vi "DRIVE_STRAIGHT_CAM.vi"(10 "argv":string[](array[string]), 11 "args":u8) -> ()   [LabVIEW 2011]
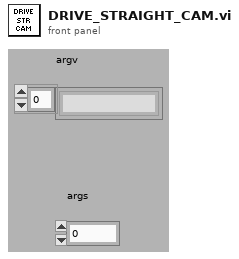
[diagram p1: front panel]
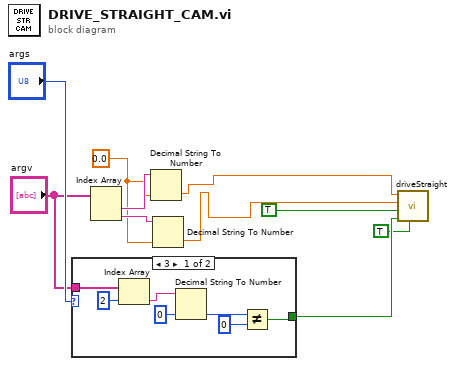
[diagram p0: block diagram]
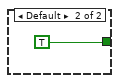
[diagram p2: hidden frame]
diagram:
  w8 = 0.0
  n1 = case shown="3" "args" {
    tunnel: "argv" -> [w17 _]
    tunnel: [w13 TRUE ("Do Speed Control?")] -> w2
    frame 3 {
      n2 = Index Array(array=w17, index=2) -> (element=w15:string)
      n3 = Decimal String To Number(string=w15, default (0L)=0 ("default (0 I32)")) -> (number=w12:i32)  [unwired: 1 in, 1 out]
      n4 = Not Equal?(x=w12, y=0) -> (x != y?=w13:bool)
    }
    frame Default {
    }
  }
  n5 = Index Array(array="argv") -> (element #1=w10:string, element #2=w9:string)  [unwired: 2 in]
  n6 = Decimal String To Number(string=w10, default (0L)=w8) -> (number=w7:dbl)  [unwired: 1 in, 1 out]
  n7 = Decimal String To Number(string=w9, default (0L)=w8) -> (number=w6:dbl)  [unwired: 1 in, 1 out]
  n8 = call "driveStraight.vi"("Use Camera"=TRUE, "Reset Encoders"=w2, "Do Speed Control?"=TRUE, "Speed (ft/sec)"=w6, "Distance"=w7) -> ()  [unwired: 7 in]
